vi "keithley_6510_iv_continuous_reading1.vi"() -> ()   [LabVIEW 2019]
panel:
  out "output array":dbl[][](array[numeric])
  out "concatenated string":string
  out "current":dbl[](graph)
  in  "stop":bool
  out "read buffer 2":string
  out "voltage":dbl[](graph)
  out "read buffer":string
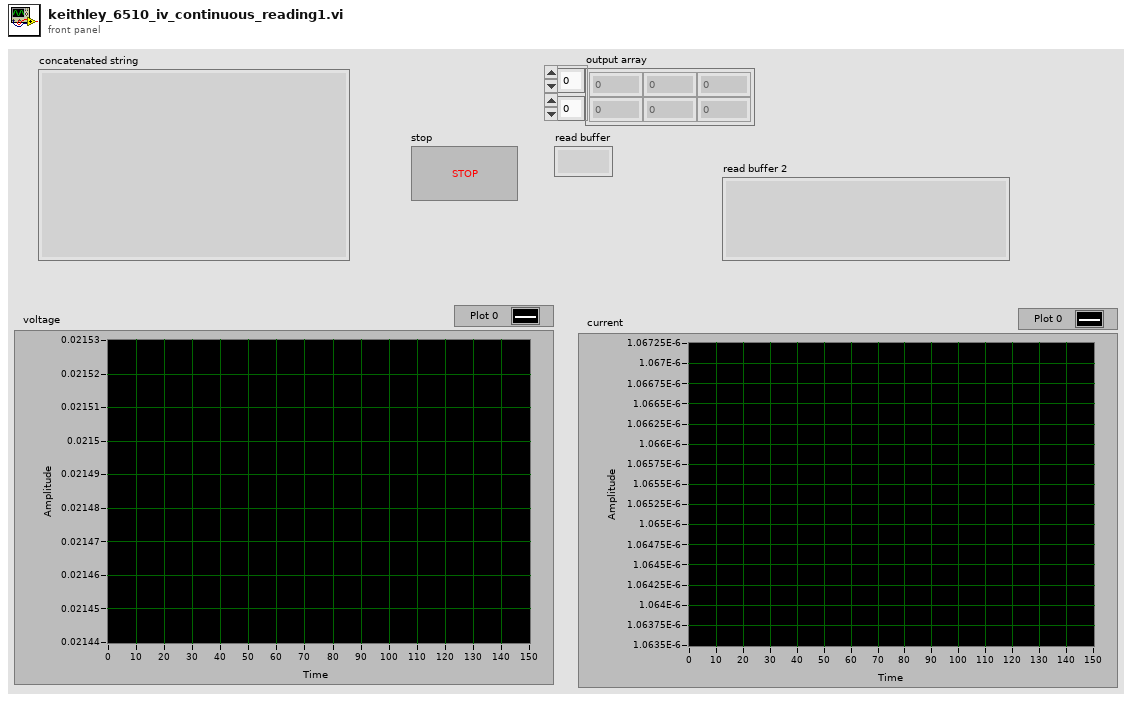
[diagram p1: front panel]
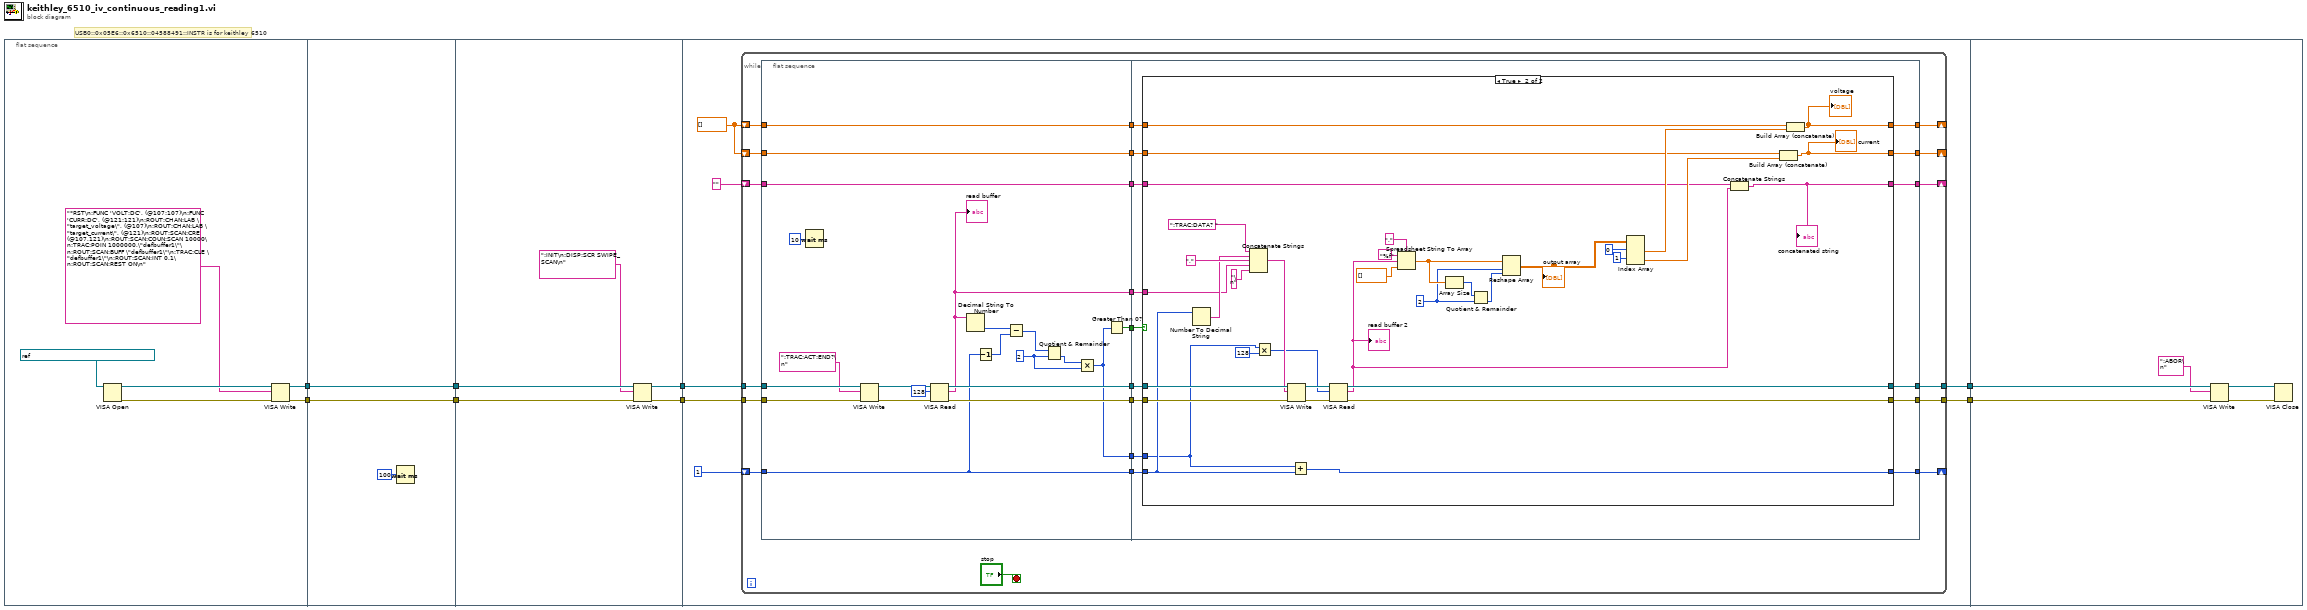
[diagram p0: block diagram]
diagram:
  # "USB0::0x05E6::0x6510::04588491::INSTR is for keithley 6510"
  n1 = flat-sequence {
    tunnel: [w11] -> w8
    tunnel: [w10] -> w7
    tunnel: w8 -> [w16]
    tunnel: w7 -> [w15]
    tunnel: [w16] -> w6
    tunnel: [w15] -> w5
    tunnel: w6 -> [w22]
    tunnel: w5 -> [w21]
    tunnel: [w19] -> w4
    tunnel: [w18] -> w3
    tunnel: w4 -> [w29]
    tunnel: w3 -> [w28]
    tunnel: [w27] -> w2
    tunnel: [w26] -> w1
    tunnel: w2 -> [w134]
    tunnel: w1 -> [w133]
    frame #0 {
      n2 = VISA Open(VISA resource name=refnum<visa-resource-name> "USB0::0x05E6::0x6510::04588491::INSTR") -> (VISA resource name=w13:refnum<visa-resource-name>, error out=w12:errorcluster)  [unwired: 4 in]
      n3 = VISA Write(VISA resource name=w13, write buffer="*RST\n:FUNC 'VOLT:DC', (@107:107)\n:FUNC 'CURR:DC', (@121:121)\n:ROUT:CHAN:LAB \"target_voltage\", (@107)\n:ROUT:CHAN:LAB \"target_current\", (@121)\n:ROUT:SCAN:CRE (@107,121)\n:ROUT:SCAN:COUN:SCAN 10000\n:TRAC:POIN 1000000,\"defbuffer1\"\n:ROUT:SCAN:BUFF \"defbuffer1\"\n:TRAC:CLE \"defbuffer1\"\n:ROUT:SCAN:INT 0.1\n:ROUT:SCAN:REST ON\n", error in (no error)=w12) -> (VISA resource name out=w11:refnum<visa-resource-name>, error out=w10:errorcluster)  [unwired: 1 out]
    }
    frame #1 {
      n4 = Wait (ms)(milliseconds to wait=u32 100) -> ()  [unwired: 1 out]
    }
    frame #2 {
      n5 = VISA Write(VISA resource name=w22, write buffer=":INIT\n:DISP:SCR SWIPE_SCAN\n", error in (no error)=w21) -> (VISA resource name out=w19:refnum<visa-resource-name>, error out=w18:errorcluster)  [unwired: 1 out]
    }
    frame #3 {
      w24 = dbl[] [] ("array type (2D Dbl)")
      n6 = while {
        tunnel: w29 -> [w50]
        tunnel: w28 -> [w49]
        tunnel: [w48] -> w27
        tunnel: [w47] -> w26
        shift-right: [w41] -> _
        shift-left: 1 -> [w43]
        shift-right: [w36] -> _
        shift-left: w24 -> [w38]
        shift-right: [w33] -> _
        shift-left: w24 -> [w35]
        shift-right: [w30] -> _
        shift-left: "" ("string") -> [w32]
        stop <- "stop" stop-if-true
        n7 = flat-sequence {
          tunnel: w50 -> [w72]
          tunnel: w49 -> [w71]
          tunnel: [w67] -> w46
          tunnel: [w66] -> w45
          tunnel: [w57] -> w44
          tunnel: w43 -> [w61]
          tunnel: [w61] -> w42
          tunnel: [w60] -> w40
          tunnel: [w52] -> w39
          tunnel: w38 -> [w63]
          tunnel: [w63] -> w37
          tunnel: w35 -> [w62]
          tunnel: [w62] -> w34
          tunnel: w32 -> [w53]
          tunnel: [w53] -> w31
          tunnel: [w84] -> w47
          tunnel: [w85] -> w48
          tunnel: w46 -> [w87]
          tunnel: w45 -> [w86]
          tunnel: w44 -> [w83]
          tunnel: w42 -> [w82]
          tunnel: [w81] -> w41
          tunnel: w40 -> [w80]
          tunnel: w39 -> [w79]
          tunnel: w37 -> [w78]
          tunnel: [w77] -> w36
          tunnel: w34 -> [w76]
          tunnel: [w75] -> w33
          tunnel: w31 -> [w74]
          tunnel: [w73] -> w30
          frame #0 {
            w54 = 2 ("y")
            n8 = Wait (ms)(milliseconds to wait=u32 10) -> ()  [unwired: 1 out]
            n9 = VISA Write(VISA resource name=w72, write buffer=":TRAC:ACT:END?\n", error in (no error)=w71) -> (VISA resource name out=w70:refnum<visa-resource-name>, error out=w69:errorcluster)  [unwired: 1 out]
            n10 = VISA Read(VISA resource name=w70, byte count=u32 128, error in (no error)=w69) -> (VISA resource name out=w67:refnum<visa-resource-name>, read buffer=w60:string, error out=w66:errorcluster)  [unwired: 1 out]
            "read buffer" <- w60
            n11 = Decimal String To Number(string=w60) -> (number=w59:i32)  [unwired: 2 in, 1 out]
            n12 = Decrement(x=w61) -> (x-1=w58:i32)
            n13 = Subtract(x=w59, y=w58) -> (x-y=w56:i32)
            n14 = Quotient & Remainder(x=w56, y=w54) -> (floor(x/y)=w55:i32)  [unwired: 1 out]
            n15 = Multiply(x=w55, y=w54) -> (x*y=w52:i32)
            n16 = Greater Than 0?(x=w52) -> (x > 0?=w57:bool)
          }
          frame #1 {
            n17 = case shown="True" w83 {
              tunnel: w87 -> [w93 w127]
              tunnel: w86 -> [w92 w126]
              tunnel: [w93 w122] -> w85
              tunnel: [w92 w121] -> w84
              tunnel: w82 -> [w91 w119]
              tunnel: [w91 w117] -> w81
              tunnel: w80 -> [_ w116]
              tunnel: w79 -> [_ w114]
              tunnel: w78 -> [w90 w109]
              tunnel: [w90 w108] -> w77
              tunnel: w76 -> [w89 w106]
              tunnel: [w89 w104] -> w75
              tunnel: w74 -> [w88 w99]
              tunnel: [w88 w97] -> w73
              frame False {
              }
              frame True {
                w101 = 2 ("dimension size")
                n18 = Number To Decimal String(number=w119) -> (decimal integer string=w118:string)  [unwired: 1 in]
                n19 = Concatenate Strings(":TRAC:DATA? " ("string"), w118, "," ("string"), w116, "\n" ("string")) -> (w125:string)
                n20 = Multiply(x=w114, y=128) -> (x*y=w113:i32)
                n21 = VISA Write(VISA resource name=w127, write buffer=w125, error in (no error)=w126) -> (VISA resource name out=w124:refnum<visa-resource-name>, error out=w123:errorcluster)  [unwired: 1 out]
                n22 = Add(x=w114, y=w119) -> (x+y=w117:i32)
                n23 = VISA Read(VISA resource name=w124, byte count=w113, error in (no error)=w123) -> (VISA resource name out=w122:refnum<visa-resource-name>, read buffer=w98:string, error out=w121:errorcluster)  [unwired: 1 out]
                "read buffer 2" <- w98
                n24 = Spreadsheet String To Array(delimiter (Tab)=",", format string="%f", spreadsheet string=w98, array type (2D Dbl)=dbl[] []) -> (array=w103:dbl[])
                n25 = Array Size(array=w103) -> (size(s)=w102:i32)
                n26 = Quotient & Remainder(x=w102, y=w101) -> (floor(x/y)=w100:i32)  [unwired: 1 out]
                n27 = Reshape Array(w103, w101, w100) -> (w96:dbl[][])
                "output array" <- w96
                n28 = Index Array(array=w96, index (row) #1=0 ("index (row)"), index (row) #2=1 ("index (row)")) -> (element #1=w107:dbl[], element #2=w105:dbl[])  [unwired: 2 in]
                n29 = Concatenate Strings(w99, w98) -> (w97:string)
                "concatenated string" <- w97
                n30 = Build Array (concatenate)(w106, w105) -> (w104:dbl[])
                "current" <- w104
                n31 = Build Array (concatenate)(w109, w107) -> (w108:dbl[])
                "voltage" <- w108
              }
            }
          }
        }
      }
    }
    frame #4 {
      n32 = VISA Write(VISA resource name=w134, write buffer=":ABOR\n", error in (no error)=w133) -> (VISA resource name out=w132:refnum<visa-resource-name>, error out=w131:errorcluster)  [unwired: 1 out]
      n33 = VISA Close(VISA resource name=w132, error in (no error)=w131) -> ()  [unwired: 1 out]
    }
  }
